vi "TTA_MXG_CW.vi"(0 "VISA resource In":refnum<visa-resource-name>, 5 "Frequency (MHz)":dbl, 7 "Output Power\nLevel (dBm)":dbl, 11 "error in":errorcluster) -> (4 "VISA resource Out":refnum<visa-resource-name>, 15 "error out":errorcluster)   [LabVIEW 2016]
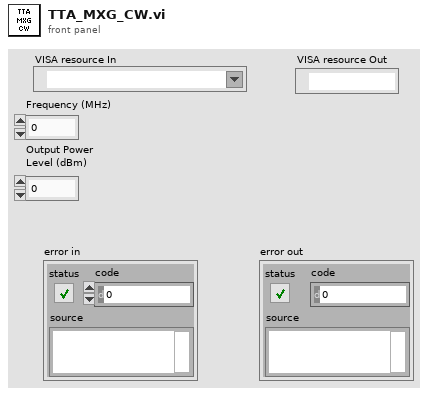
[diagram p1: front panel]
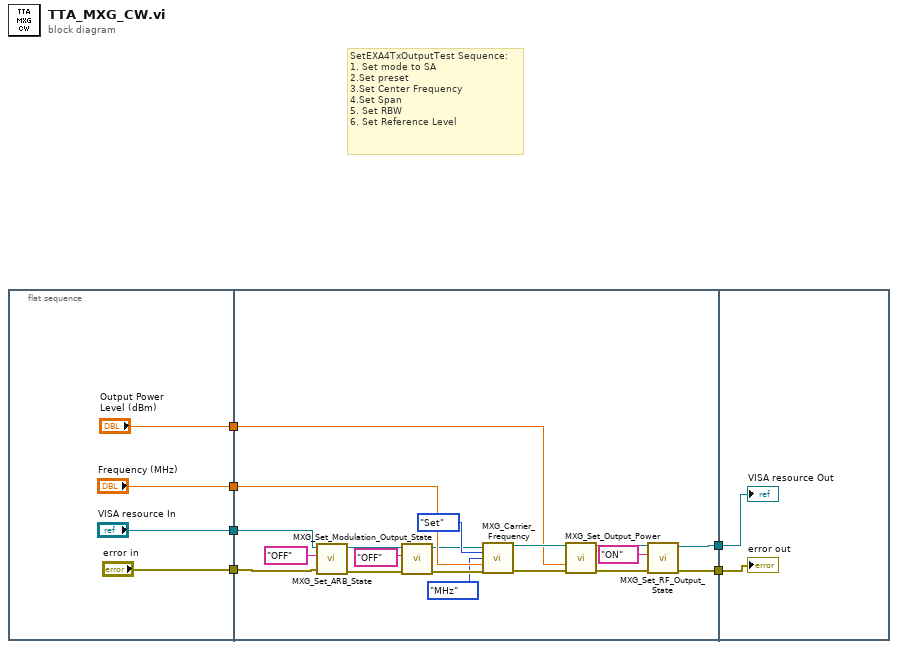
[diagram p0: block diagram]
diagram:
  # "SetEXA4TxOutputTest Sequence:\n1. Set mode to SA\n2.Set preset\n3.Set Center Frequency\n4.Set Span\n5. Set RBW\n6. Set Reference Level"
  n1 = flat-sequence {
    tunnel: ["error in"] -> w6
    tunnel: ["VISA resource In"] -> w5
    tunnel: ["Frequency (MHz)"] -> w4
    tunnel: ["Output Power\nLevel (dBm)"] -> w2
    tunnel: w6 -> [w28]
    tunnel: w5 -> [w27]
    tunnel: w4 -> [w22]
    tunnel: [w12] -> w3
    tunnel: w2 -> [w17]
    tunnel: [w11] -> w1
    tunnel: w3 -> [w31]
    tunnel: w1 -> [w30]
    frame #0 {
    }
    frame #1 {
      n2 = call "MXG_Set_ARB_State.vi"("error in"=w28, "ARB State"="OFF", "VISA resource name"=w27) -> ("error out"=w26:errorcluster, "VISA resource name"=w24:refnum<visa-resource-name>)  [unwired: 7 in]
      n3 = call "MXG_Set_Modulation_Output_State.vi"("error in"=w26, "Modulation State"="OFF", "VISA resource name"=w24) -> ("error out"=w23:errorcluster, "VISA resource name"=w19:refnum<visa-resource-name>)  [unwired: 7 in]
      n4 = call "MXG_Carrier_Frequency.vi"("VISA resource name"=w19, "Mode"=enum16{"Set", "Get"}."Set", "Units"=enum16{"Hz", "kHz", "MHz", "GHz"}."MHz", "Frequency"=w22, "error in"=w23) -> ("VISA resource name"=w18:refnum<visa-resource-name>, "error out"=w16:errorcluster)  [unwired: 8 in, 1 out]
      n5 = call "MXG_Set_Output_Power.vi"("VISA resource name"=w18, "Output Power\nLevel (dBm)"=w17, "error in"=w16) -> ("VISA resource name"=w15:refnum<visa-resource-name>, "error out"=w14:errorcluster)  [unwired: 11 in]
      n6 = call "MXG_Set_RF_Output_State.vi"("error in"=w14, "RF Output State"="ON", "VISA resource name"=w15) -> ("error out"=w11:errorcluster, "VISA resource name"=w12:refnum<visa-resource-name>)  [unwired: 7 in]
    }
    frame #2 {
      "VISA resource Out" <- w31
      "error out" <- w30
    }
  }
